vi "Read Array of Voltages.vi"(8 "error in (no error)":errorcluster, 11 "Galvo in":refnum<class "Galvo.lvclass">) -> (0 "error out":errorcluster, 2 "Array of Voltages":dbl[][](array[numeric]), 3 "Galvo out":refnum<class "Galvo.lvclass">)   [LabVIEW 2015, in "Galvo.lvclass"]
uses:
  Galvo.lvclass
  Galvo.lvclass/Galvo.ctl
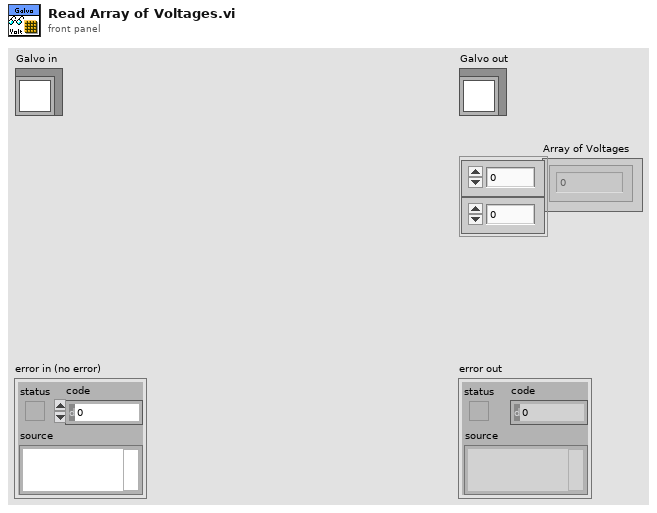
[diagram p1: front panel]
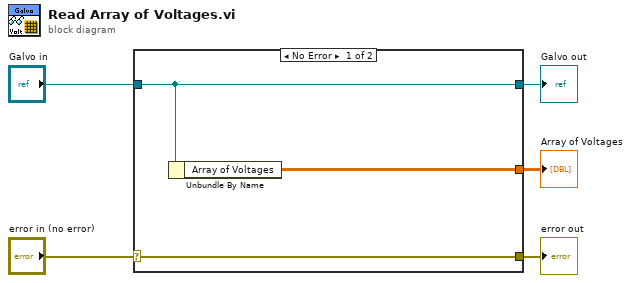
[diagram p0: block diagram]
diagram:
  n1 = case shown="No Error" "error in (no error)" {
    selector: "error in (no error)" -> [w8 w9]
    tunnel: [w8 w9] -> w4
    tunnel: [w7 w10] -> w2
    tunnel: "Galvo in" -> [w7 w10]
    tunnel: [w6 _] -> w1
    frame No Error {
      n2 = Unbundle By Name(w7) -> ("Array of Voltages"=w6:dbl[][])
    }
    frame Error {
    }
  }
  "error out" <- w4
  "Galvo out" <- w2
  "Array of Voltages" <- w1
